vi "2xK2200s_OFF.vi"() -> ()   [LabVIEW 2014]
uses:
  C:/Users/rad/Desktop/Keithley 2200 Series Power Supplies Ver 1.2 (LV2009)/Keithley 2200 Series/Keithley 2200 Series.lvlib
panel:
  in  "VISA resource name 2":refnum<visa-resource-name>
  in  "VISA resource name":refnum<visa-resource-name>
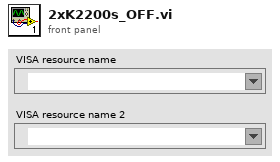
[diagram p1: front panel]
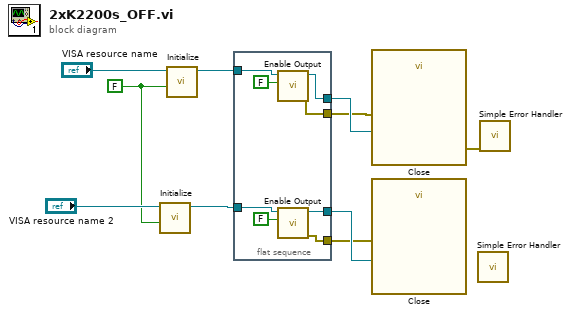
[diagram p0: block diagram]
diagram:
  w1 = FALSE ("Reset (True)")
  n1 = call "Initialize.vi"("Reset (True)"=w1, "VISA resource name"="VISA resource name 2") -> ("VISA resource name out"=w4:refnum<visa-resource-name>)  [unwired: 8 in, 1 out]
  n2 = call "Initialize.vi"("Reset (True)"=w1, "VISA resource name"="VISA resource name") -> ("VISA resource name out"=w5:refnum<visa-resource-name>)  [unwired: 8 in, 1 out]
  n3 = flat-sequence {
    tunnel: w5 -> [w17]
    tunnel: w4 -> [w15]
    tunnel: [w14] -> w9
    tunnel: [w13] -> w6
    tunnel: [w12] -> w7
    tunnel: [w11] -> w8
    frame #0 {
      n4 = call "Enable Output.vi"("Enable Output (T: Enable)"=FALSE, "VISA resource name"=w17) -> ("error out"=w13:errorcluster, "VISA resource name out"=w14:refnum<visa-resource-name>)  [unwired: 1 in, 7 out]
      n5 = call "Enable Output.vi"("Enable Output (T: Enable)"=FALSE, "VISA resource name"=w15) -> ("error out"=w12:errorcluster, "VISA resource name out"=w11:refnum<visa-resource-name>)  [unwired: 1 in, 7 out]
    }
  }
  n6 = call "Close.vi"("error in (no error)"=w6, "VISA resource name"=w9) -> ("error out"=w10:errorcluster)  [unwired: 9 in]
  n7 = call "Close.vi"("error in (no error)"=w7, "VISA resource name"=w8) -> ()  [unwired: 9 in, 1 out]
  n8 = call <vilib>:"Simple Error Handler.vi"() -> ()  [unwired: 5 in, 5 out]
  n9 = call <vilib>:"Simple Error Handler.vi"("error in (no error)"=w10) -> ()  [unwired: 4 in, 5 out]
